vi "fp1task1.vi"() -> ()   [LabVIEW 2016]
uses:
  <vilib>/NXT/Subs/ColorSensorColors.ctl
  <vilib>/NXT/Block Support/NXT_ButtonSelector.ctl
  <vilib>/NXT/Block Support/NXT_InputPort.ctl
  <vilib>/NXT/Block Support/NXT_OutputPort.ctl
  <vilib>/NXT/Dual Mode Library/Waits/Wait_Btn.vi
  <vilib>/NXT/NXTIO Xnodes/NXTIONodeSubVIs/NXTMotorRunDistance.vi
  <vilib>/NXT/Dual Mode Library/Waits/Wait_Num.vi
  <vilib>/NXT/Dual Mode Library/Sensors/EV3_Color_Color.vi
  <vilib>/NXT/NXTIO Xnodes/AddressXNode/NXTIOAddress.xnode
  <vilib>/NXT/NXTIO Xnodes/NXTIOXNode/NXTIO.xnode
  <vilib>/NXT/Subs/LVHSConnector.ctl
  <vilib>/NXT/LegoClasses/BrickReference/BrickReference.lvclass
  <vilib>/Analysis/NI_AALBase.lvlib
panel:
  out "Detected Color":T1
  out "standard deviation DC":dbl format="%0.2f"
  out "mean DC":dbl format="%0.2f"
  out "Detected Color":T1[](array[typedef])
  out "Detected Color Number":u32[](array[numeric])
  out "standard deviation SV":dbl format="%0.2f"
  out "mean SV":dbl format="%0.2f"
  out "Reflected Scaled Value":dbl[](array[numeric])
  out "Reflected Scaled Value":sgl
  # "ENGR 111\n\nSection 423\n \nTeam 12\n\nResults for flash project 4  testing on table"
  # "By submitting this assignment, I agree to the following:\n“Aggies do not lie, cheat, or steal, or tolerate those who do”\n“I have not given or received any unauthorized aid on this assignment”\n\nName:   Ericka Reyes\nSection:  423\nTeam:  12\nAssignment: fp1task1\nDate:  12 11 2017"
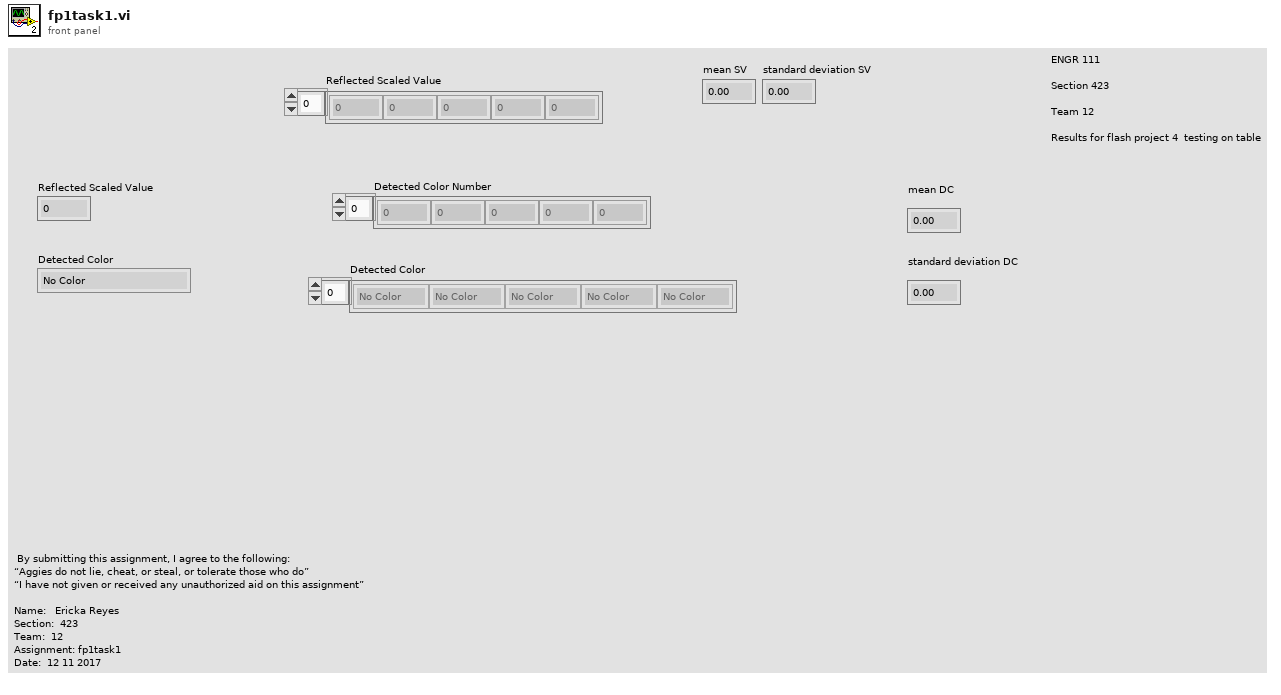
[diagram p1: front panel]
types:
  T1 = typedef "ColorSensorColors.ctl" = enum16{"No Color", "Black", "Blue", "Green", "Yellow", "Red", "White", "Brown"}
  T2 = typedef "NXT_ButtonSelector.ctl" = u16
  T3 = typedef "LVHSConnector.ctl" = refnum<class "BrickReference.lvclass">
  T4 = typedef "NXT_OutputPort.ctl" = u8
  T5 = typedef "NXT_InputPort.ctl" = u32
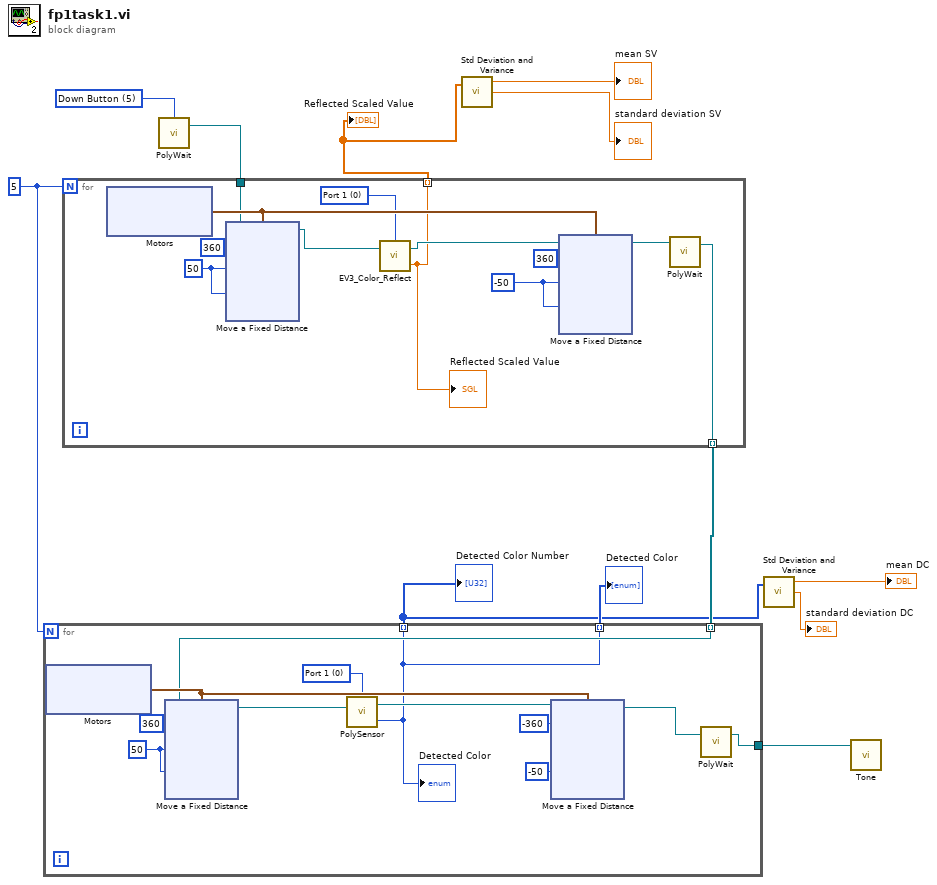
[diagram p0: block diagram]
diagram:
  w2 = 5
  w10 = T2 5 items=["Enter button"=3, "Left button"=2, "Right button"=1, "Up Button"=4, "Down Button"=5] ("Button (Enter button)")
  n1 = call-poly <vilib>:"PolyWait.vi"("Button (Enter button)"=w10) -> ("NXT/EV3"=w9:T3)  [unwired: 3 in]
  n2 = for {
    N: w2 -> [_]
    tunnel: [w16] -> w12 mode=indexing
    tunnel: w9 -> [w15]
    tunnel: [w13] -> w1 mode=indexing
    w14 = T5 0 items=["Port 1", "Port 2", "Port 3", "Port 4"] ("Port (Port 1)")
    w20 = i8 -50 ("Speed 1")
    w21 = 360 ("Distance 1")
    w23 = i8 50 ("Speed 1")
    w24 = 360 ("Distance 1")
    n3 = xnode "Motors"() -> ("Motor"=w22:cluster{"Port":T4, "Port":T4})
    n4 = xnode "Move a Fixed Distance"("Speed 2"=w23, "Speed 1"=w23, "Distance 2"=w24, "Distance 1"=w24, "Motors"=w22, "NXT/EV3"=w15) -> ("NXT/EV3"=w19:T3)
    n5 = call <vilib>:"EV3_Color_Reflect.vi"("NXT/EV3"=w19, "Port (Port 1)"=w14) -> ("Scaled Value"=w13:sgl, "NXT/EV3"=w18:T3)  [unwired: 1 in]
    "Reflected Scaled Value" <- w13
    n6 = xnode "Move a Fixed Distance"("Speed 2"=w20, "Speed 1"=w20, "Distance 2"=w21, "Distance 1"=w21, "Motors"=w22, "NXT/EV3"=w18) -> ("NXT/EV3"=w17:T3)
    n7 = call-poly <vilib>:"PolyWait.vi"("NXT/EV3"=w17) -> ("NXT/EV3"=w16:T3)  [unwired: 3 in]
  }
  "Reflected Scaled Value" <- w1
  n8 = for {
    N: w2 -> [_]
    tunnel: w12 -> [w54] mode=indexing
    tunnel: [w55] -> w11
    tunnel: [w50] -> w3 mode=indexing
    tunnel: [w50] -> w4 mode=indexing
    w53 = T5 0 items=["Port 1", "Port 2", "Port 3", "Port 4"] ("Port (Port 1)")
    w57 = i8 -50 ("Speed 2")
    w58 = -360 ("Distance 1")
    w60 = i8 50 ("Speed 1")
    w61 = 360 ("Distance 1")
    n9 = xnode "Motors"() -> ("Motor"=w59:cluster{"Port":T4, "Port":T4})
    n10 = xnode "Move a Fixed Distance"("Speed 2"=w60, "Speed 1"=w60, "Distance 2"=w61, "Distance 1"=w61, "Motors"=w59, "NXT/EV3"=w54) -> ("NXT/EV3"=w52:T3)
    n11 = call-poly <vilib>:"PolySensor.vi"("NXT/EV3"=w52, "Port (Port 1)"=w53) -> ("Detected Color"=w50:T1, "NXT/EV3"=w51:T3)  [unwired: 1 in]
    "Detected Color" <- w50
    n12 = xnode "Move a Fixed Distance"("Speed 2"=w57, "Speed 1"=w57, "Distance 2"=w58, "Distance 1"=w58, "Motors"=w59, "NXT/EV3"=w51) -> ("NXT/EV3"=w56:T3)
    n13 = call-poly <vilib>:"PolyWait.vi"("NXT/EV3"=w56) -> ("NXT/EV3"=w55:T3)  [unwired: 3 in]
  }
  "Detected Color Number" <- w3
  "Detected Color" <- w4
  n14 = call <vilib>:"Std Deviation and Variance.vi"("X"=w1) -> ("mean"=→"mean SV":dbl, "standard deviation"=→"standard deviation SV":dbl)  [unwired: 1 in, 1 out]
  n15 = call <vilib>:"Std Deviation and Variance.vi"("X"=w3) -> ("mean"=→"mean DC":dbl, "standard deviation"=→"standard deviation DC":dbl)  [unwired: 1 in, 1 out]
  n16 = call <vilib>:"Tone.vi"("NXT/EV3"=w11) -> ()  [unwired: 3 in, 1 out]
